vi "Overview Cursor Release.vi"(8 "error in":errorcluster, 11 "XYGraphOverview in":refnum<class "XYGraphOverview.lvclass">) -> (0 "error out":errorcluster, 3 "XYGraphOverview out":refnum<class "XYGraphOverview.lvclass">)   [LabVIEW 2020, in "XYGraphOverview.lvlib" / "XYGraphOverview.lvclass"]
uses:
  XYGraphOverview.lvclass
  XYGraphOverview.lvclass/XYGraphOverview.ctl
  Read Block Color.vi
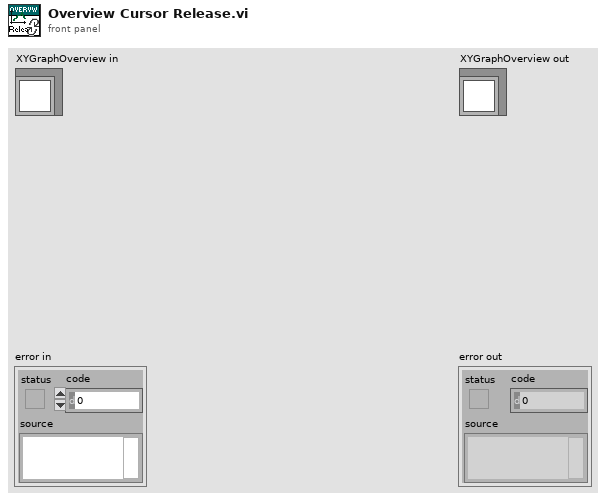
[diagram p1: front panel]
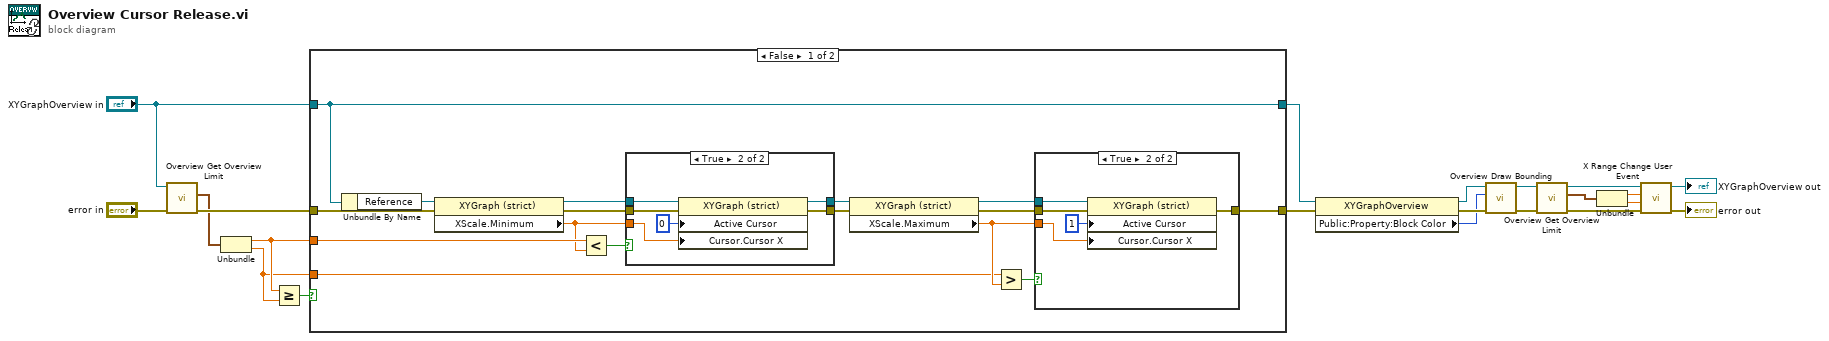
[diagram p0: block diagram]
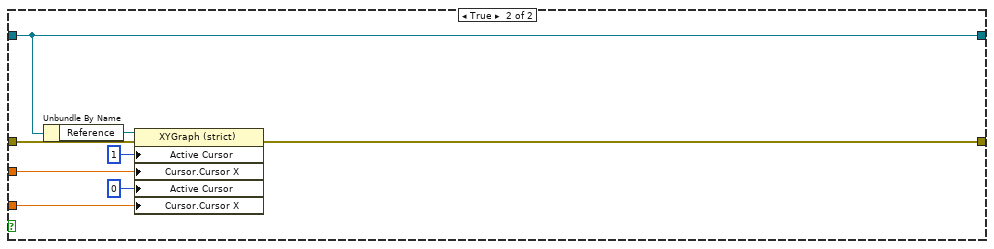
[diagram p4: hidden frame]
diagram:
  n1 = call "Overview Get Overview Limit.vi"("error in"="error in", "XYGraphOverview in"="XYGraphOverview in") -> ("error out"=w18:errorcluster, "Limit"=w17:cluster{"Lower Limit":dbl, "Upper Limit":dbl})  [unwired: 7 in, 1 out]
  n2 = Unbundle(w17) -> ("Lower Limit"=w16:dbl, "Upper Limit"=w15:dbl)
  n3 = Greater Or Equal?(x=w16, y=w15) -> (x >= y?=w21:bool)
  n4 = case shown="False" w21 {
    tunnel: w18 -> [w37 w59]
    tunnel: w15 -> [w25 w57]
    tunnel: w16 -> [w36 w54]
    tunnel: [w24 w55] -> w4
    tunnel: "XYGraphOverview in" -> [w23 w53]
    tunnel: [w23 w53] -> w3
    frame False {
      n5 = Unbundle By Name(w23) -> ("Reference"=w22:refnum<vi>)
      n6 = property on="Property Node" class="XYGraph (strict)"(reference=w22, error in=w37) -> (reference out=w33:refnum<vi>, error out=w32:errorcluster, "XScale.Minimum"=w34:dbl)
      n7 = Less?(x=w36, y=w34) -> (x < y?=w35:bool)
      n8 = case shown="True" w35 {
        tunnel: w32 -> [w45 w51]
        tunnel: w33 -> [w44 w50]
        tunnel: w34 -> [_ w48]
        tunnel: [w45 w47] -> w27
        tunnel: [w44 w46] -> w26
        frame False {
        }
        frame True {
          n9 = property class="XYGraph (strict)"(reference=w50, error in=w51, "Active Cursor"=u32 0, "Cursor.Cursor X"=w48) -> (reference out=w46:refnum<vi>, error out=w47:errorcluster)
        }
      }
      n10 = property on="Property Node" class="XYGraph (strict)"(reference=w26, error in=w27) -> (reference out=w30:refnum<vi>, error out=w31:errorcluster, "XScale.Maximum"=w29:dbl)
      n11 = Greater?(x=w25, y=w29) -> (0:w28:bool)
      n12 = case shown="True" w28 {
        tunnel: w31 -> [w38 w43]
        tunnel: w30 -> [_ w42]
        tunnel: w29 -> [_ w40]
        tunnel: [w38 w39] -> w24
        frame False {
        }
        frame True {
          n13 = property class="XYGraph (strict)"(reference=w42, error in=w43, "Active Cursor"=u32 1, "Cursor.Cursor X"=w40) -> (error out=w39:errorcluster)  [unwired: 1 out]
        }
      }
    }
    frame True {
      n14 = Unbundle By Name(w53) -> ("Reference"=w52:refnum<vi>)
      n15 = property class="XYGraph (strict)"(reference=w52, error in=w59, "Active Cursor"=u32 1, "Cursor.Cursor X"=w54, "Active Cursor"=u32 0, "Cursor.Cursor X"=w57) -> (error out=w55:errorcluster)  [unwired: 1 out]
    }
  }
  n16 = property class="XYGraphOverview"(reference=w3, error in=w4) -> (reference out=w6:refnum<class "XYGraphOverview.lvclass">, error out=w7:errorcluster, "Public:Property:Block Color"=w5:u32)
  n17 = call "Overview Draw Bounding.vi"("error in (no error)"=w7, "Color"=w5, "XYGraphOverview in"=w6) -> ("error out"=w14:errorcluster, "XYGraphOverview out"=w13:refnum<class "XYGraphOverview.lvclass">)  [unwired: 7 in]
  n18 = call "Overview Get Overview Limit.vi"("error in"=w14, "XYGraphOverview in"=w13) -> ("error out"=w10:errorcluster, "Limit"=w12:cluster{"Lower Limit":dbl, "Upper Limit":dbl}, "XYGraphOverview out"=w11:refnum<class "XYGraphOverview.lvclass">)  [unwired: 7 in]
  n19 = Unbundle(w12) -> ("Lower Limit"=w9:dbl, "Upper Limit"=w8:dbl)
  n20 = call "X Range Change User Event.vi"("error in (no error)"=w10, "Upper Range"=w8, "Lower Range"=w9, "XYGraphOverview in"=w11) -> ("error out"=→"error out":errorcluster, "XYGraphOverview out"=→"XYGraphOverview out":refnum<class "XYGraphOverview.lvclass">)  [unwired: 6 in]
